vi "Read Main Refs.vi"(8 "error in (no error)":errorcluster, 11 "HGF_Application in":refnum<class "HGF_Application.lvclass">) -> (0 "error out":errorcluster, 1 "Status Info Queue":refnum<queue>, 2 "Main Stop Event":refnum<user-event>, 3 "HGF_Application out":refnum<class "HGF_Application.lvclass">, 4 "Navigation Sub Panel":refnum<vi>, 5 "Info Event":refnum<class "HGF_Event.lvclass">, 6 "Application Sub Panel":refnum<vi>, 7 "Main Menu":refnum<k9>)   [LabVIEW 2012, in "HGF_ApplicationBaseClasses.lvlib" / "HGF_Application.lvclass"]
uses:
  HGF_Application.lvclass
  HGF_BaseClasses/HGF_Event/HGF_Event.lvclass
  HGF_Application.lvclass/HGF_Application.ctl
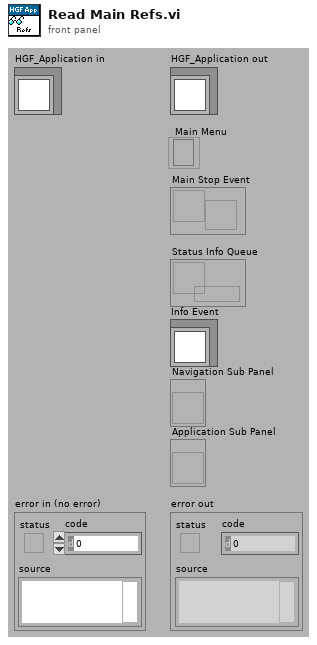
[diagram p1: front panel]
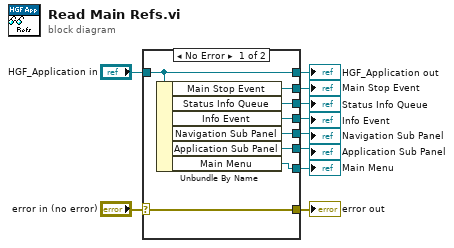
[diagram p0: block diagram]
diagram:
  n1 = case shown="No Error" "error in (no error)" {
    selector: "error in (no error)" -> [w18 w19]
    tunnel: [w18 w19] -> w9
    tunnel: [w17 w20] -> w7
    tunnel: "HGF_Application in" -> [w17 w20]
    tunnel: [w16 _] -> w6
    tunnel: [w15 _] -> w5
    tunnel: [w14 _] -> w4
    tunnel: [w13 _] -> w3
    tunnel: [w12 _] -> w2
    tunnel: [w11 _] -> w1
    frame No Error {
      n2 = Unbundle By Name(w17) -> ("Main Stop Event"=w16:refnum<user-event>, "Status Info Queue"=w15:refnum<queue>, "Info Event"=w14:refnum<class "HGF_Event.lvclass">, "Navigation Sub Panel"=w13:refnum<vi>, "Application Sub Panel"=w12:refnum<vi>, "Main Menu"=w11:refnum<k9>)
    }
    frame Error {
    }
  }
  "error out" <- w9
  "HGF_Application out" <- w7
  "Main Stop Event" <- w6
  "Status Info Queue" <- w5
  "Info Event" <- w4
  "Navigation Sub Panel" <- w3
  "Application Sub Panel" <- w2
  "Main Menu" <- w1
